vi "Configure Trigger (General).vi"(0 "VISA resource name":refnum<visa-resource-name>, 7 "Holdoff Time (2E-8 s)":dbl=2e-08, 9 "Trigger Mode (0: Auto)":i32(ring) items=["Auto", "Normal"], 11 "error in (no error)":errorcluster) -> (4 "VISA resource name out":refnum<visa-resource-name>, 15 "error out":errorcluster)   [LabVIEW 2017, in "Scope.lvlib" / "Tektronix DPO MSO 2000 4000 Series.lvlib"]
doc: "Configures holdoff time and trigger mode of the A trigger."
uses:
  Tektronix DPO MSO 2000 4000 Series.lvlib
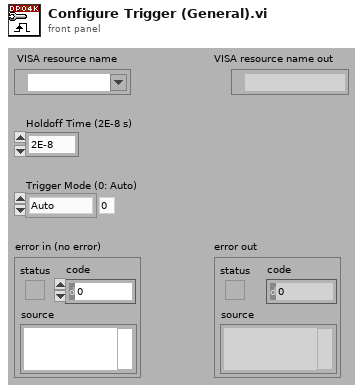
[diagram p1: front panel]
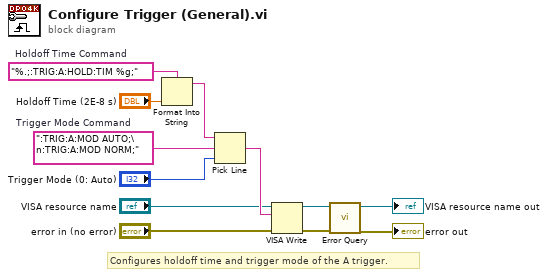
[diagram p0: block diagram]
diagram:
  w10 = ":TRIG:A:MOD AUTO;\n:TRIG:A:MOD NORM;"  # Trigger Mode Command
  w12 = "%.;:TRIG:A:HOLD:TIM %g;"  # Holdoff Time Command
  # "Configures holdoff time and trigger mode of the A trigger."
  n1 = Format Into String(format string=w12, "Holdoff Time (2E-8 s)") -> (resulting string=w8:string)  [unwired: 2 in, 1 out]
  n2 = Pick Line(string ("")=w8, multi-line string=w10, line index="Trigger Mode (0: Auto)") -> (output string=w7:string)
  n3 = VISA Write(VISA resource name="VISA resource name", write buffer=w7, error in (no error)="error in (no error)") -> (VISA resource name out=w4:refnum<visa-resource-name>, error out=w3:errorcluster)  [unwired: 1 out]
  n4 = call "Error Query.vi"("error in (no error)"=w3, "VISA resource name"=w4) -> ("error out"=→"error out":errorcluster, "VISA resource name out"=→"VISA resource name out":refnum<visa-resource-name>)  [unwired: 6 in, 2 out]
